vi "Powermeter module.vi"(0 "instrument handle":refnum<visa-resource-name>, 5 "Average Time (0.0)":dbl=0.1, 7 "Wavelength":dbl=930.0 caption="Wavelength (0.0)", 9 "Enum":T1, 11 "error in (no error)":errorcluster {"code" format="%.0x"}) -> (4 "instrument handle 2":refnum<visa-resource-name>, 6 "Average Time":dbl, 8 "Wavelength":dbl, 10 "Sensor Name":string, 15 "error out":errorcluster)   [LabVIEW 2018]
uses:
  Controls/Powermeter Actions.ctl
panel:
  out "Power":dbl
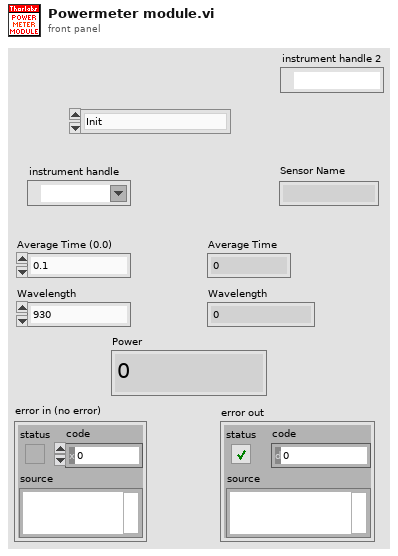
[diagram p1: front panel]
types:
  T1 = typedef "Powermeter Actions.ctl" = enum16{"Init", "Set-Get Avg", "Set-Get Wavelength", "Do measure"}
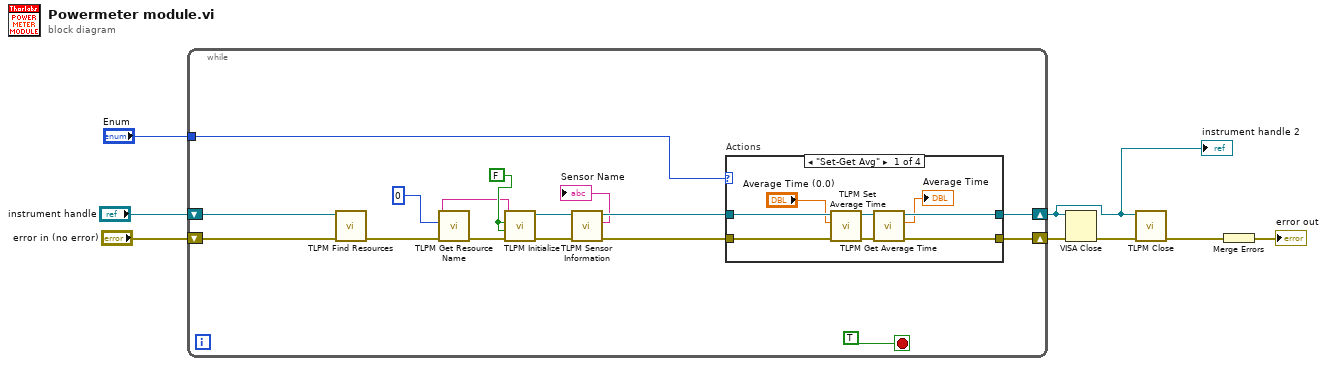
[diagram p0: block diagram]
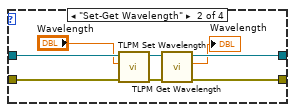
[diagram p2: hidden frame]
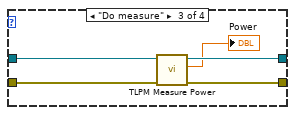
[diagram p3: hidden frame]
diagram:
  n1 = while {
    shift-right: [w19] -> w4
    shift-left: "error in (no error)" -> [w22]
    tunnel: "Enum" -> [w17]
    shift-right: [w20] -> w3
    shift-left: "instrument handle" -> [w23]
    stop <- TRUE stop-if-true
    w10 = FALSE ("ID Query (Do Query)")
    n2 = call "TLPM Find Resources.vi"("error in (no error)"=w22, "instrument handle"=w23) -> ("error out"=w14:errorcluster)  [unwired: 7 in, 2 out]
    n3 = call "TLPM Get Resource Name.vi"("error in (no error)"=w14, "Index (0)"=u32 0) -> ("error out"=w12:errorcluster, "Resource Name"=w9:string)  [unwired: 7 in, 1 out]
    n4 = call "TLPM Initialize.vi"("error in (no error)"=w12, "Reset Device (Reset Device)"=w10, "ID Query (Do Query)"=w10, "resource name"=w9) -> ("error out"=w11:errorcluster, "instrument handle out"=w13:refnum<visa-resource-name>)  [unwired: 6 in]
    n5 = call "TLPM Sensor Information.vi"("error in (no error)"=w11, "instrument handle"=w13) -> ("error out"=w21:errorcluster, "Sensor Name"=→"Sensor Name":string, "instrument handle out"=w18:refnum<visa-resource-name>)  [unwired: 2 in, 5 out]
    n6 = case "Actions" shown="\"Set-Get Avg\"" w17 {
      tunnel: w18 -> [w32 w40 w45 w46]
      tunnel: w21 -> [w31 w35 w42 w47]
      tunnel: [w27 w38 w44 w46] -> w20
      tunnel: [w28 w33 w41 w47] -> w19
      frame "Set-Get Avg" {
        n7 = call "TLPM Set Average Time.vi"("error in (no error)"=w31, "Average Time (0.0)"="Average Time (0.0)", "instrument handle"=w32) -> ("error out"=w29:errorcluster, "instrument handle out"=w30:refnum<visa-resource-name>)  [unwired: 7 in]
        n8 = call "TLPM Get Average Time.vi"("error in (no error)"=w29, "instrument handle"=w30) -> ("error out"=w28:errorcluster, "Average Time"=→"Average Time":dbl, "instrument handle out"=w27:refnum<visa-resource-name>)  [unwired: 7 in]
      }
      frame "Set-Get Wavelength" {
        n9 = call "TLPM Set Wavelength.vi"("error in (no error)"=w35, "Wavelength (0.0)"="Wavelength", "instrument handle"=w40) -> ("error out"=w34:errorcluster, "instrument handle out"=w39:refnum<visa-resource-name>)  [unwired: 7 in]
        n10 = call "TLPM Get Wavelength.vi"("error in (no error)"=w34, "instrument handle"=w39) -> ("error out"=w33:errorcluster, "Wavelength"=→"Wavelength":dbl, "instrument handle out"=w38:refnum<visa-resource-name>)  [unwired: 7 in]
      }
      frame "Do measure" {
        n11 = call "TLPM Measure Power.vi"("error in (no error)"=w42, "instrument handle"=w45) -> ("error out"=w41:errorcluster, "Power"=→"Power":dbl, "instrument handle out"=w44:refnum<visa-resource-name>)  [unwired: 7 in]
      }
      frame "Init", Default {
      }
    }
  }
  "instrument handle 2" <- w3
  n12 = VISA Close(VISA resource name=w3, error in (no error)=w4) -> (error out=w2:errorcluster)
  n13 = call "TLPM Close.vi"("error in (no error)"=w2, "instrument handle"=w3) -> ("error out"=w1:errorcluster)  [unwired: 9 in]
  n14 = Merge Errors(w1) -> (→"error out":errorcluster)
